vi "Get TDMS File Groups and Channels.vi"(8 "error in":errorcluster, 11 "TDMS ref in":refnum<k34>) -> (0 "error out":errorcluster, 2 "file contents":cluster{string, string[]}[](array[cluster]), 3 "TDMS ref out":refnum<k34>)   [LabVIEW 2020, in "NI_TDMS File Viewer.lvlib"]
uses:
  <vilib>/Utility/TDMS File Viewer/NI_TDMS File Viewer.lvlib
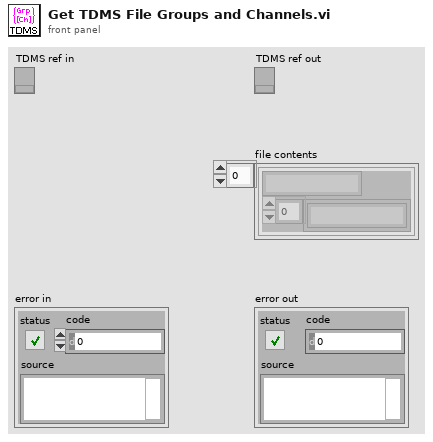
[diagram p1: front panel]
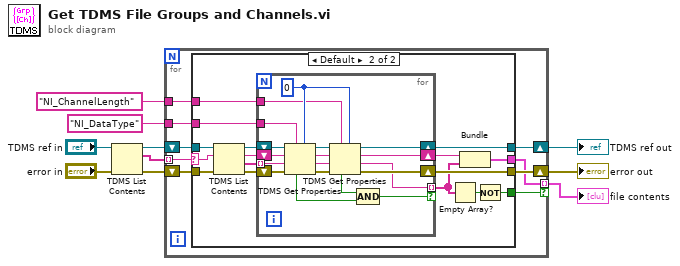
[diagram p0: block diagram]
diagram:
  n1 = TDMS List Contents(4:"error in", 7:"TDMS ref in") -> (0:w9:errorcluster, 2:w3:string[], 3:w2:refnum<k34>)  [unwired: 1 in, 1 out]
  n2 = for {
    tunnel: w3 -> [w17] mode=indexing
    shift-right: [w15] -> w4
    shift-left: w2 -> [w16]
    shift-right: [w18] -> w10
    shift-left: w9 -> [w19]
    tunnel: [w13] -> w5 mode=indexing if=w14
    tunnel: "NI_ChannelLength" ("property name") -> [w12]
    tunnel: "NI_DataType" ("property name") -> [w11]
    n3 = case shown="Default" w17 {
      selector: w17 -> [_ w34]
      tunnel: w16 -> [w20 w33]
      tunnel: [w20 w28] -> w15
      tunnel: w19 -> [w21 w37]
      tunnel: [w21 w35] -> w18
      tunnel: [_ w31] -> w14
      tunnel: [_ w30] -> w13
      tunnel: w12 -> [_ w24]
      tunnel: w11 -> [_ w23]
      frame "" {
      }
      frame Default {
        n4 = TDMS List Contents(4:w37, 6:w34, 7:w33) -> (0:w36:errorcluster, 1:w26:string[], 2:w27:string, 3:w29:refnum<k34>)
        n5 = for {
          shift-right: [w41] -> w28
          shift-left: w29 -> [w52]
          shift-right: [w53] -> w35
          shift-left: w36 -> [w55]
          tunnel: w26 -> [w50] mode=indexing
          shift-right: [w46] -> w25
          shift-left: w27 -> [w51]
          tunnel: [w45] -> w22 mode=indexing if=w38
          tunnel: w24 -> [w43]
          tunnel: w23 -> [w42]
          w44 = u16 0
          n6 = TDMS Get Properties(5:w44, 7:w42, 8:w55, 9:w50, 10:w51, 11:w52) -> (0:w54:errorcluster, 1:w48:string, 2:w49:string, 3:w47:refnum<k34>, 6:w39:bool)  [unwired: 1 out]
          n7 = TDMS Get Properties(5:w44, 7:w43, 8:w54, 9:w48, 10:w49, 11:w47) -> (0:w53:errorcluster, 1:w45:string, 2:w46:string, 3:w41:refnum<k34>, 6:w40:bool)  [unwired: 1 out]
          n8 = Compound Arithmetic op=AND(w40, w39) -> (w38:bool)
        }
        n9 = Empty Array?(array=w22) -> (empty?=w32:bool)
        n10 = Bundle(w25, w22) -> (w30:cluster{string, string[]})  [unwired: 1 in]
        n11 = Not(x=w32) -> (.not. x?=w31:bool)
      }
    }
  }
  "error out" <- w10
  "file contents" <- w5
  "TDMS ref out" <- w4
